vi "create_data_folder.vi"(8 "error in (no error)":errorcluster, 10 "Experiment description suffix":string, 11 "General Data Files Path":path=path "C:/Users/QCC/Documents/Cesium_project/LabVIEW Projects/data") -> (0 "error out":errorcluster, 3 "Specific Data Files Path":path)   [LabVIEW 2013]
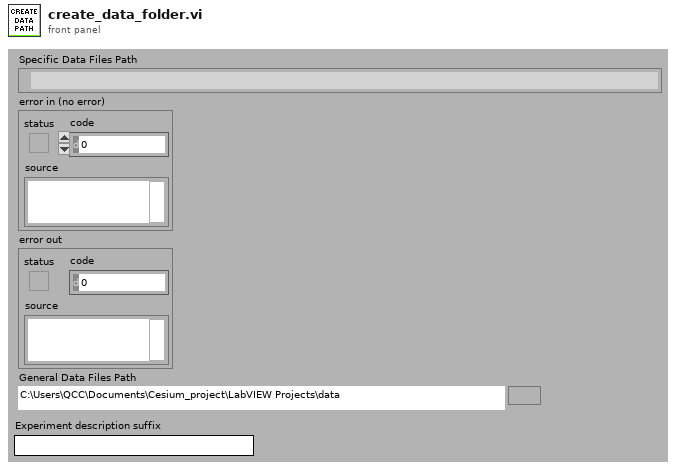
[diagram p1: front panel]
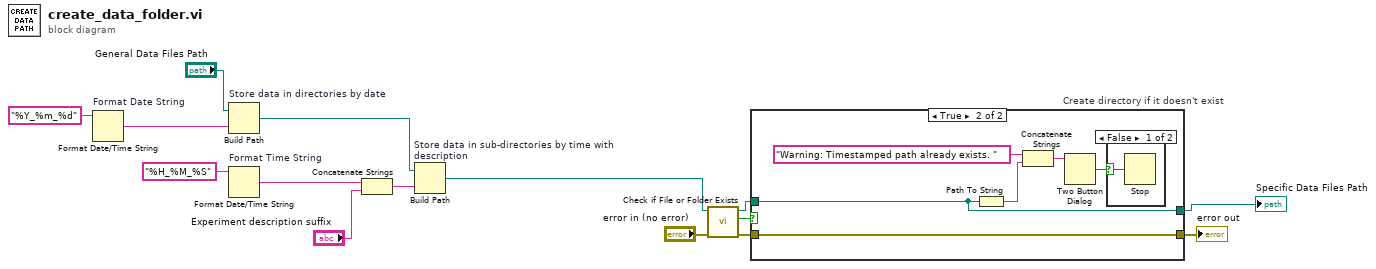
[diagram p0: block diagram]
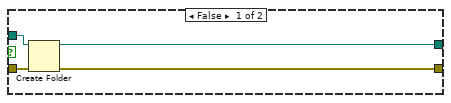
[diagram p2: hidden frame]
diagram:
  n1 = Format Date/Time String "Format Date String"(time format string (%c)="%Y_%m_%d") -> (date/time string=w14:string)  [unwired: 2 in]
  n2 = Build Path "Store data in directories by date"(base path="General Data Files Path", name or relative path=w14) -> (appended path=w7:path)
  n3 = Format Date/Time String "Format Time String"(time format string (%c)="%H_%M_%S") -> (date/time string=w2:string)  [unwired: 2 in]
  n4 = Concatenate Strings(w2, "Experiment description suffix") -> (w1:string)
  n5 = Build Path "Store data in sub-directories by time with description"(base path=w7, name or relative path=w1) -> (appended path=w6:path)
  n6 = call <vilib>:"Check if File or Folder Exists.vi"("error in (no error)"="error in (no error)", "path"=w6) -> ("error out"=w11:errorcluster, "file or folder exists?"=w10:bool, "dup path"=w9:path)  [unwired: 7 in]
  n7 = case "Create directory if it doesn't exist" shown="True" w10 {
    tunnel: w11 -> [w19 w25]
    tunnel: [w18 w25] -> w5
    tunnel: w9 -> [w16 w24]
    tunnel: [w17 w24] -> w4
    frame False {
      n8 = Create Folder(path (use dialog)=w16, error in=w19) -> (created path=w17:path, error out=w18:errorcluster)  [unwired: 1 in, 1 out]
    }
    frame True {
      n9 = Path To String(path=w24) -> (string=w22:string)
      n10 = Concatenate Strings("Warning: Timestamped path already exists. " ("string"), w22) -> (w23:string)
      n11 = Two Button Dialog(message=w23) -> (T button?=w20:bool)  [unwired: 2 in]
      n12 = case shown="False" w20 {
        selector: w20 -> [w26 _]
        frame False {
          n13 = Stop(stop? (T)=w26) -> ()
        }
        frame True {
        }
      }
    }
  }
  "error out" <- w5
  "Specific Data Files Path" <- w4
